vi "Chart Property Node.vi"() -> ()   [LabVIEW 2015]
panel:
  in  "stop":bool
  in  "Chart Mode":enum16{"Sweep", "Scope", "Strip"}(ring)
  out "Under Range":bool
  out "Over Range":bool
  out "Chart":dbl(graph)
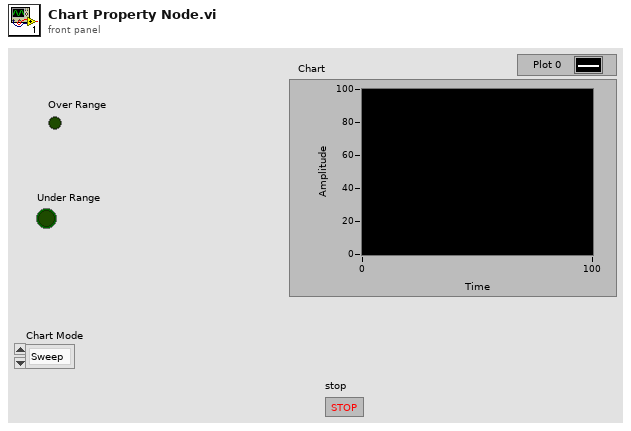
[diagram p1: front panel]
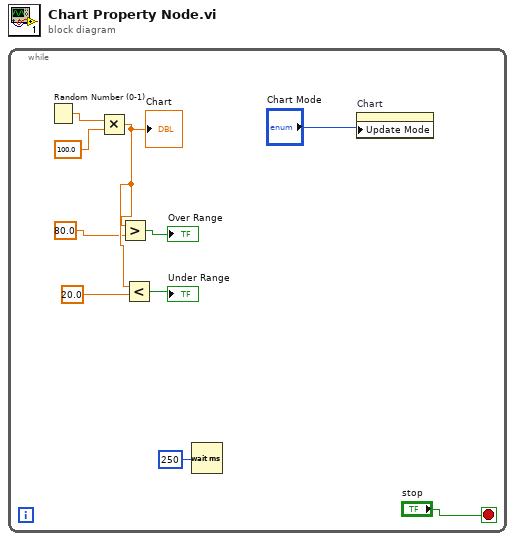
[diagram p0: block diagram]
diagram:
  n1 = while {
    stop <- "stop" stop-if-true
    n2 = Random Number (0-1)() -> (number: 0 to 1=w9:dbl)
    n3 = Multiply(x=w9, y=100.0) -> (x*y=w6:dbl)
    "Chart" <- w6
    n4 = Greater?(x=w6, y=80.0) -> (0:→"Over Range":bool)
    n5 = Less?(x=w6, y=20.0) -> (x < y?=→"Under Range":bool)
    n6 = Wait (ms)(milliseconds to wait=250) -> ()  [unwired: 1 out]
    n7 = property on="Chart" class="WFChart (strict)"("Update Mode"="Chart Mode") -> ()  [unwired: 2 in, 2 out]
  }
